vi "CreateListener.vi"(8 "error in (no error)":errorcluster, 11 "Qbus in":refnum<class "Qbus.lvclass">) -> (0 "error out":errorcluster, 3 "Qbus out":refnum<class "Qbus.lvclass">)   [LabVIEW 2017, in "ServerComm.lvlib"]
doc: "Integrates the Server Comm process with the Qbus message bus."
uses:
  <vilib>/addons/InsightCM/Devices/Shared/Common/ServerComm/ServerComm.lvlib
  <vilib>/addons/Qbus/Qbus.lvclass
  <vilib>/addons/InsightCM/Devices/Shared/Common/TracePointSynchronizer/TracePointSynchronizer.lvlib
  <vilib>/addons/InsightCM/Devices/Shared/Common/USBDrive/USBDrive.lvlib
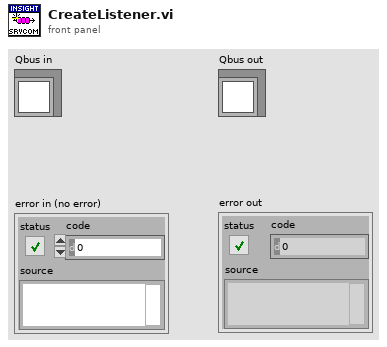
[diagram p1: front panel]
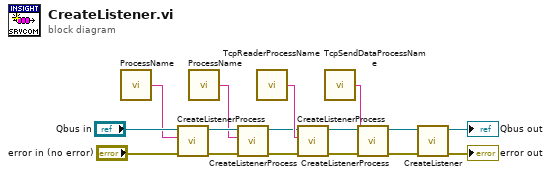
[diagram p0: block diagram]
diagram:
  n1 = call <vilib>:"ProcessName.vi"() -> ("process name"=w14:string)  [unwired: 5 in]
  n2 = call <vilib>:"CreateListenerProcess.vi"("error in (no error)"="error in (no error)", "process name"=w14, "Qbus in"="Qbus in") -> ("error in (no error)"=w6:errorcluster, "Qbus out"=w7:refnum<class "Qbus.lvclass">)  [unwired: 7 in]
  n3 = call <vilib>:"ProcessName.vi"() -> ("ProcessName"=w5:string)  [unwired: 5 in]
  n4 = call <vilib>:"CreateListenerProcess.vi"("error in (no error)"=w6, "process name"=w5, "Qbus in"=w7) -> ("error in (no error)"=w9:errorcluster, "Qbus out"=w8:refnum<class "Qbus.lvclass">)  [unwired: 7 in]
  n5 = call <vilib>:"TcpReaderProcessName.vi"() -> ("process name"=w11:string)  [unwired: 5 in]
  n6 = call <vilib>:"CreateListenerProcess.vi"("error in (no error)"=w9, "process name"=w11, "Qbus in"=w8) -> ("error in (no error)"=w13:errorcluster, "Qbus out"=w12:refnum<class "Qbus.lvclass">)  [unwired: 7 in]
  n7 = call <vilib>:"TcpSendDataProcessName.vi"() -> ("process name"=w10:string)  [unwired: 5 in]
  n8 = call <vilib>:"CreateListenerProcess.vi"("error in (no error)"=w13, "process name"=w10, "Qbus in"=w12) -> ("error in (no error)"=w2:errorcluster, "Qbus out"=w4:refnum<class "Qbus.lvclass">)  [unwired: 7 in]
  n9 = call <vilib>:"CreateListener.vi"("error in (no error)"=w2, "Qbus in"=w4) -> ("error out"=→"error out":errorcluster, "Qbus out"=→"Qbus out":refnum<class "Qbus.lvclass">)  [unwired: 8 in]
